vi "Simulated Values.vi"() -> ()   [LabVIEW 2020, in "Simulated Interlocks.lvclass"]
uses:
  Simulated Interlocks/Simulated Interlocks.lvclass
  Door Interlocks/Interlock Values.ctl
  Door Interlocks/Mode of Operation.ctl
  Door Interlocks/Door Interlocks.lvclass
panel:
  in  "Interlock Values":T1
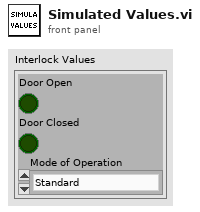
[diagram p1: front panel]
types:
  T1 = typedef "Door Interlocks.lvclass/Interlock Values.ctl" = cluster{"Door Open":bool, "Door Closed":bool, "Mode of Operation":T2}
  T2 = typedef "Door Interlocks.lvclass/Mode of Operation.ctl" = enum16{"Standard", "Interlock Override"}
diagram:
